vi "Parse_Parameter.vi"(8 "error in (no error)":errorcluster, 9 "Parameter In":T1, 10 "ItemName":i32, 11 "Value (String)":string) -> (0 "error out":errorcluster, 1 "Parameter Out":T1)   [LabVIEW 2019]
uses:
  XML_Parameter.ctl
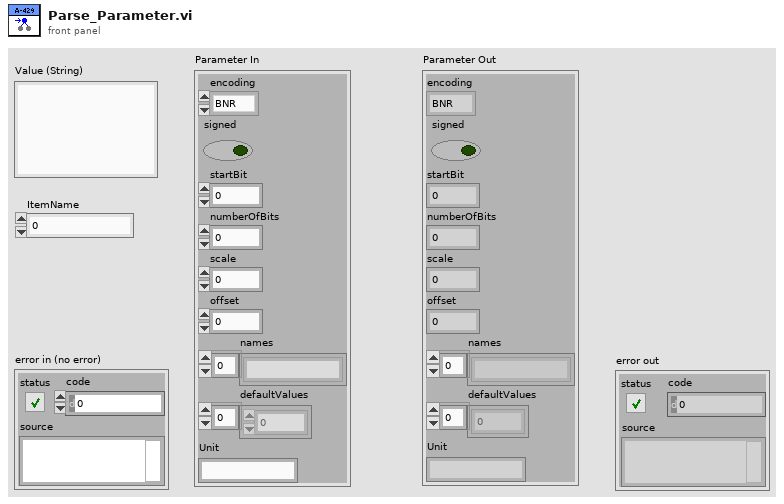
[diagram p1: front panel]
types:
  T1 = typedef "XML_Parameter.ctl" = cluster{"encoding":enum16{"BNR", "BCD", "Discrete"}, "signed":bool, "startBit":i32, "numberOfBits":i32, "scale":dbl, "offset":dbl, "names":string[], "defaultValues":dbl[], "Unit":string}
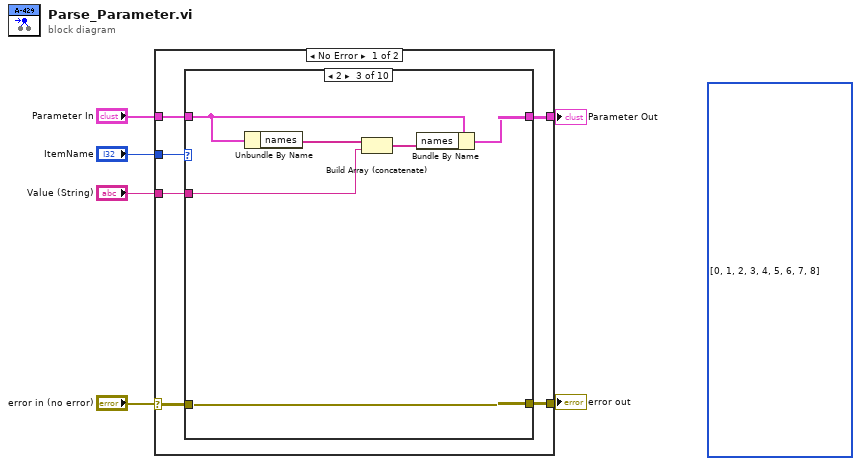
[diagram p0: block diagram]
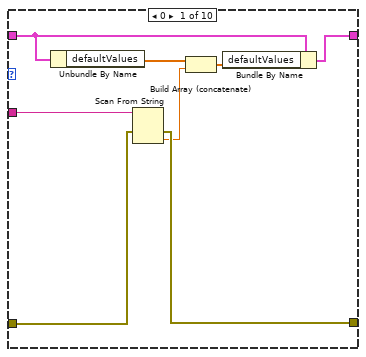
[diagram p2: hidden frame]
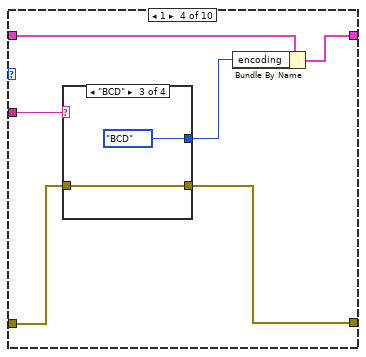
[diagram p4: hidden frame]
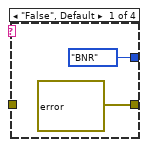
[diagram p5: hidden frame]
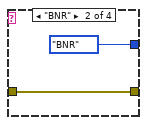
[diagram p6: hidden frame]
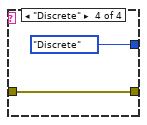
[diagram p7: hidden frame]
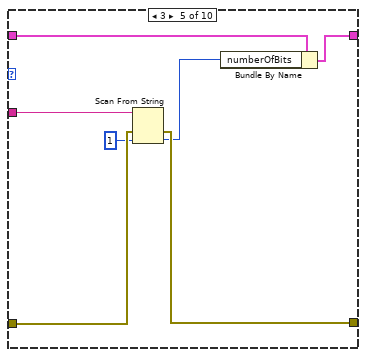
[diagram p8: hidden frame]
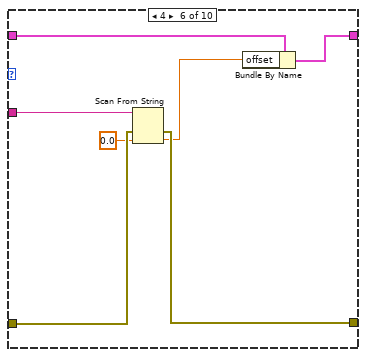
[diagram p9: hidden frame]
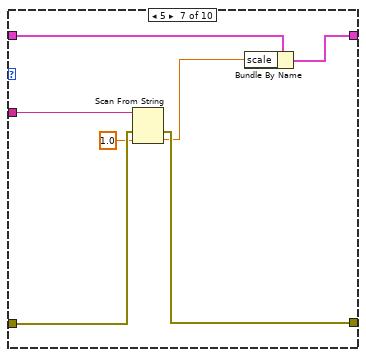
[diagram p10: hidden frame]
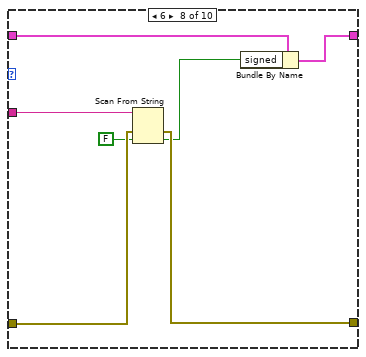
[diagram p11: hidden frame]
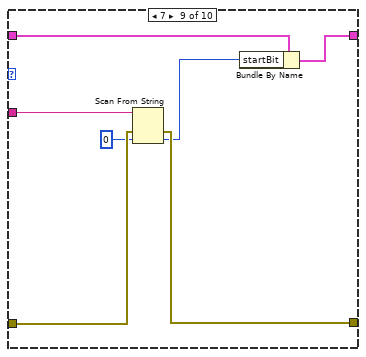
[diagram p12: hidden frame]
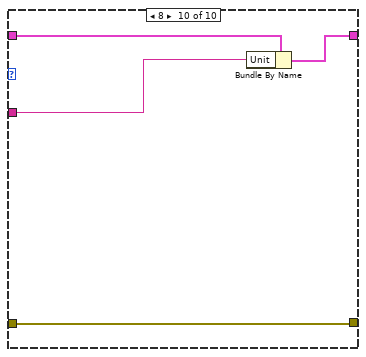
[diagram p13: hidden frame]
diagram:
  (unwired) i32[] [0, 1, 2, 3, 4, 5, 6, 7, 8] items=["defaultValue", "encoding", "name", "numberOfBits", "offset", "scale", "signed", "startBit", "unit"] ("ItemsElementName")
  n1 = case shown="No Error" "error in (no error)" {
    selector: "error in (no error)" -> [w9 w83]
    tunnel: [w8 w83] -> w5
    tunnel: "Parameter In" -> [w11 w82]
    tunnel: [w7 w82] -> w3
    tunnel: "ItemName" -> [w12 _]
    tunnel: "Value (String)" -> [w10 _]
    frame No Error {
      n2 = case shown="2" w12 {
        tunnel: w11 -> [w16 w22 w27 w33 w45 w52 w59 w66 w73 w80]
        tunnel: w10 -> [w20 _ w24 w32 w49 w56 w63 w70 w77 w79]
        tunnel: w9 -> [w19 w21 w23 w31 w48 w55 w62 w69 w76 w78]
        tunnel: [w18 w21 w23 w29 w47 w54 w61 w68 w75 w78] -> w8
        tunnel: [w17 w22 w28 w34 w46 w53 w60 w67 w74 w81] -> w7
        frame 0 {
          n3 = Unbundle By Name(w16) -> ("defaultValues"=w15:dbl[])
          n4 = Scan From String(input string=w20, error in=w19) -> (error out=w18:errorcluster, output 1=w14:dbl)  [unwired: 3 in, 2 out]
          n5 = Build Array (concatenate)(w15, w14) -> (w13:dbl[])
          n6 = Bundle By Name(cluster=w16, "defaultValues"=w13) -> (w17:T1)
        }
        frame 9, Default {
        }
        frame 2 {
          n7 = Unbundle By Name(w27) -> ("names"=w26:string[])
          n8 = Build Array (concatenate)(w26, w24) -> (w25:string[])
          n9 = Bundle By Name(cluster=w27, "names"=w25) -> (w28:T1)
        }
        frame 1 {
          n10 = case shown="\"BCD\"" w32 {
            tunnel: w31 -> [_ w37 w39 w41]
            tunnel: [enum16{"BNR", "BCD", "Discrete"}."BNR" ("encoding") enum16{"BNR", "BCD", "Discrete"}."BNR" ("encoding") enum16{"BNR", "BCD", "Discrete"}."BCD" ("encoding") enum16{"BNR", "BCD", "Discrete"}."Discrete" ("encoding")] -> w30
            tunnel: [errorcluster {"status"=TRUE, "code"=5015, "source"="Encoding setting not supported. Accepted\nvalues: BNR, BCD, Discrete."} ("error IO") w37 w39 w41] -> w29
            frame "False", Default {
            }
            frame "BNR" {
            }
            frame "BCD" {
            }
            frame "Discrete" {
            }
          }
          n11 = Bundle By Name(cluster=w33, "encoding"=w30) -> (w34:T1)
        }
        frame 3 {
          n12 = Scan From String(input string=w49, error in=w48, default 1=1) -> (error out=w47:errorcluster, output 1=w44:i32)  [unwired: 2 in, 2 out]
          n13 = Bundle By Name(cluster=w45, "numberOfBits"=w44) -> (w46:T1)
        }
        frame 4 {
          n14 = Scan From String(input string=w56, error in=w55, default 1=0.0) -> (error out=w54:errorcluster, output 1=w51:dbl)  [unwired: 2 in, 2 out]
          n15 = Bundle By Name(cluster=w52, "offset"=w51) -> (w53:T1)
        }
        frame 5 {
          n16 = Scan From String(input string=w63, error in=w62, default 1=1.0) -> (error out=w61:errorcluster, output 1=w58:dbl)  [unwired: 2 in, 2 out]
          n17 = Bundle By Name(cluster=w59, "scale"=w58) -> (w60:T1)
        }
        frame 6 {
          n18 = Scan From String(input string=w70, error in=w69, default 1=FALSE) -> (error out=w68:errorcluster, output 1=w65:bool)  [unwired: 2 in, 2 out]
          n19 = Bundle By Name(cluster=w66, "signed"=w65) -> (w67:T1)
        }
        frame 7 {
          n20 = Scan From String(input string=w77, error in=w76, default 1=0) -> (error out=w75:errorcluster, output 1=w72:i32)  [unwired: 2 in, 2 out]
          n21 = Bundle By Name(cluster=w73, "startBit"=w72) -> (w74:T1)
        }
        frame 8 {
          n22 = Bundle By Name(cluster=w80, "Unit"=w79) -> (w81:T1)
        }
      }
    }
    frame Error {
    }
  }
  "error out" <- w5
  "Parameter Out" <- w3
